vi "createVariable.vi"(0 "HGF_DSCVarManager in":refnum<class "HGF_DSCVarManager.lvclass">, 2 "shared variable name":string, 5 "error in (no error)":errorcluster) -> (14 "HGF_DSCVarManager out":refnum<class "HGF_DSCVarManager.lvclass">, 16 "shared variable":refnum<k21>, 19 "error out":errorcluster)   [LabVIEW 2012, in "HGF_DSC.lvlib" / "HGF_DSCVarManager.lvclass"]
uses:
  HGF_DSCVarManager.lvclass
  HGF_DSCVarManager.lvclass/HGF_DSCVarManager.ctl
  <vilib>/lvdsc/NI_DSC.lvlib
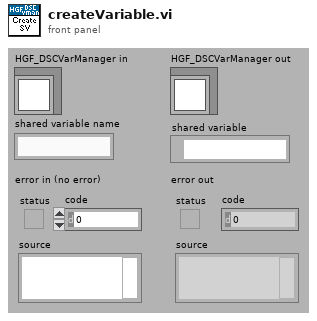
[diagram p1: front panel]
types:
  T1 = enum32{"u32BitField", "bool", "double", "string"}
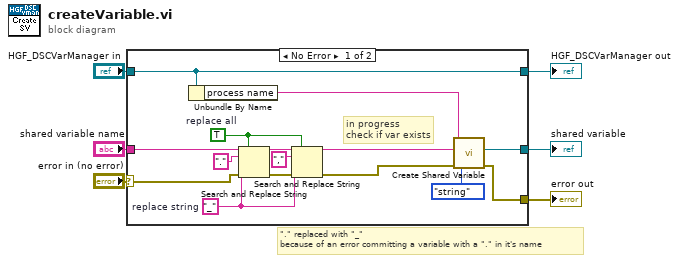
[diagram p0: block diagram]
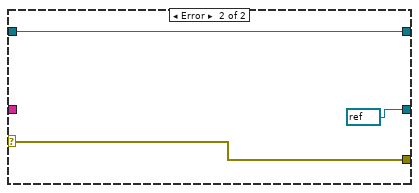
[diagram p2: hidden frame]
diagram:
  # "\".\" replaced with \"_\"\nbecause of an error committing a variable with a \".\" in it's name"
  n1 = case shown="No Error" "error in (no error)" {
    selector: "error in (no error)" -> [w15 w22]
    tunnel: [w21 w24] -> w4
    tunnel: "HGF_DSCVarManager in" -> [w21 w24]
    tunnel: "shared variable name" -> [w17 _]
    tunnel: [w19 w22] -> w2
    tunnel: [w18 refnum<k21> refnum ("shared variable")] -> w1
    frame No Error {
      w7 = TRUE  # replace all
      w8 = "_"  # replace string
      # "in progress\ncheck if var exists"
      n2 = Unbundle By Name(w21) -> ("process name"=w14:string)
      n3 = Search and Replace String(replace all?=w7, input string=w17, search string=".", replace string=w8, error in=w15) -> (result string=w13:string, error out=w12:errorcluster)  [unwired: 5 out]
      n4 = Search and Replace String(replace all?=w7, input string=w13, search string=",", replace string=w8, error in=w12) -> (result string=w10:string, error out=w11:errorcluster)  [unwired: 5 out]
      n5 = call <vilib>:"Create Shared Variable.vi"("error in (no error)"=w11, "data type"=T1."string", "shared variable name"=w10, "process name"=w14) -> ("error out"=w19:errorcluster, "shared variable"=w18:refnum<k21>)  [unwired: 2 in, 4 out]
    }
    frame Error {
    }
  }
  "error out" <- w2
  "HGF_DSCVarManager out" <- w4
  "shared variable" <- w1
